vi "Mutate System Definition Driver VI And Dependency Paths.vi"(8 "error in (no error)":errorcluster, 11 "Section Ref in":T1 format="%.0x") -> (0 "error out":errorcluster, 3 "Section Ref out":T1 format="%.0x")   [LabVIEW 2019, in "Instrument Addon System Explorer.lvlib"]
uses:
  Instrument Addon System Explorer.lvlib
  <vilib>/NI VeriStand/Custom Device API/Path Type.ctl
  <vilib>/NI VeriStand/Custom Device API/Custom Device API.lvlib
  <vilib>/NI VeriStand/Custom Device API/Path Specification.ctl
  <vilib>/NI VeriStand/Custom Device API/Custom Device Supported Target.ctl
  <vilib>/NI VeriStand/Custom Device API/Custom Device Path Data.ctl
  NationalInstruments.VeriStand.SystemDefinitionAPI
  <vilib>/NI VeriStand/Custom Device API/Custom Device Item Ref.ctl
panel:
  in  "Current Version":string
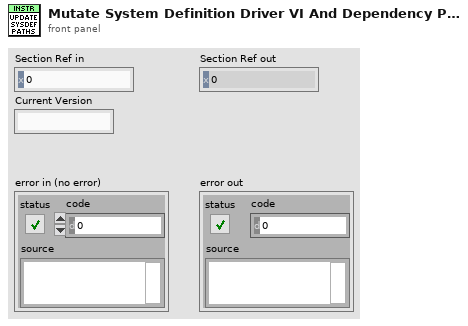
[diagram p1: front panel]
types:
  T1 = typedef "Custom Device API.lvlib/Custom Device Item Ref.ctl" = u64
  T2 = typedef "Custom Device API.lvlib/Custom Device Path Data.ctl" = cluster{"SupportedTarget":T3, "Source":T4, "RT Destination":path}
  T3 = typedef "Custom Device API.lvlib/Custom Device Supported Target.ctl" = enum16{"All", "PharLap", "VxWorks", "Windows", "Linux_32_ARM", "Linux_x64", "PharLap & Windows", "PharLap & VxWorks", "VxWorks & Windows"}
  T4 = typedef "Custom Device API.lvlib/Path Specification.ctl" = cluster{"Path":path, "Type":T5}
  T5 = typedef "Custom Device API.lvlib/Path Type.ctl" = enum16{"Absolute", "To Base", "To Common Data Dir", "To Application Data Dir"}
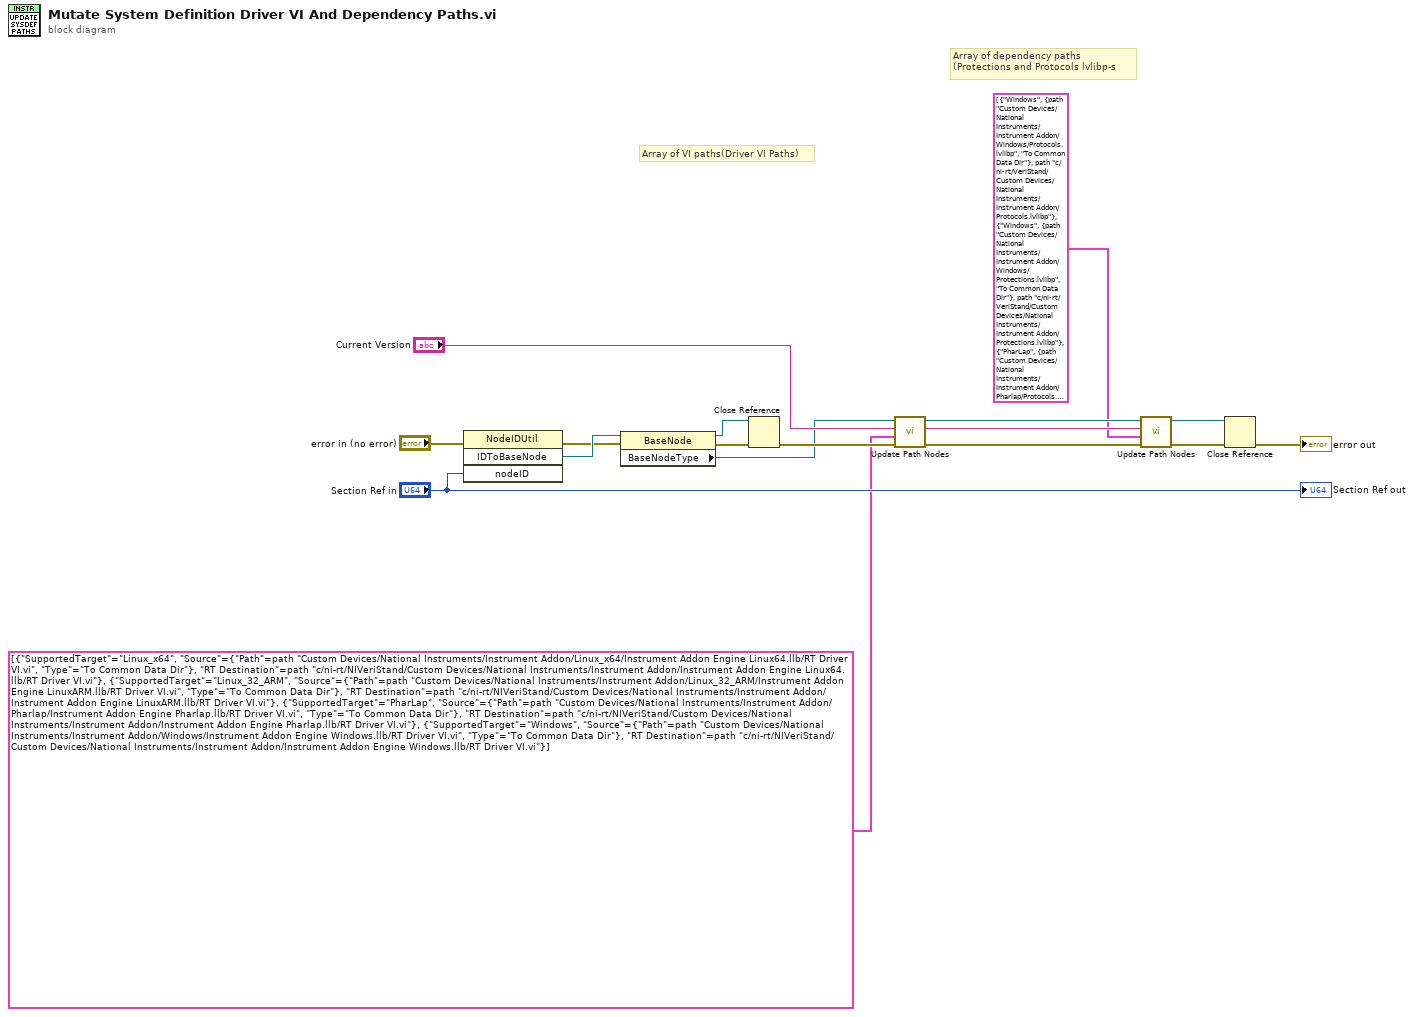
[diagram p0: block diagram]
diagram:
  # "Array of dependency paths\n(Protections and Protocols lvlibp-s"
  # "Array of VI paths(Driver VI Paths)"
  n1 = invoke class="NodeIDUtil" method="IDToBaseNode"(error in="error in (no error)", "nodeID"="Section Ref in") -> (error out=w11:errorcluster, "IDToBaseNode"=w12:refnum<k24>)  [unwired: 2 in, 2 out]
  n2 = property class="BaseNode"(reference=w12, error in=w11) -> (reference out=w14:refnum<k24>, error out=w13:errorcluster, "BaseNodeType"=w8:refnum<k24>)
  n3 = Close Reference(reference=w14, error in (no error)=w13) -> (error out=w16:errorcluster)
  n4 = call "Update Path Nodes.vi"("error in (no error)"=w16, "New Paths Array"=T2[] [{"SupportedTarget"=enum."Linux_x64", "Source"={"Path"=path "Custom Devices/National Instruments/Instrument Addon/Linux_x64/Instrument Addon Engine Linux64.llb/RT Driver VI.vi", "Type"=enum."To Common Data Dir"}, "RT Destination"=path "c:/ni-rt/NIVeriStand/Custom Devices/National Instruments/Instrument Addon/Instrument Addon Engine Linux64.llb/RT Driver VI.vi"}, {"SupportedTarget"=enum."Linux_32_ARM", "Source"={"Path"=path "Custom Devices/National Instruments/Instrument Addon/Linux_32_ARM/Instrument Addon Engine LinuxARM.llb/RT Driver VI.vi", "Type"=enum."To Common Data Dir"}, "RT Destination"=path "c:/ni-rt/NIVeriStand/Custom Devices/National Instruments/Instrument Addon/Instrument Addon Engine LinuxARM.llb/RT Driver VI.vi"}, {"SupportedTarget"=enum."PharLap", "Source"={"Path"=path "Custom Devices/National Instruments/Instrument Addon/Pharlap/Instrument Addon Engine Pharlap.llb/RT Driver VI.vi", "Type"=enum."To Common Data Dir"}, "RT Destination"=path "c:/ni-rt/NIVeriStand/Custom Devices/National Instruments/Instrument Addon/Instrument Addon Engine Pharlap.llb/RT Driver VI.vi"}, {"SupportedTarget"=enum."Windows", "Source"={"Path"=path "Custom Devices/National Instruments/Instrument Addon/Windows/Instrument Addon Engine Windows.llb/RT Driver VI.vi", "Type"=enum."To Common Data Dir"}, "RT Destination"=path "c:/ni-rt/NIVeriStand/Custom Devices/National Instruments/Instrument Addon/Instrument Addon Engine Windows.llb/RT Driver VI.vi"}] ("Driver VIs"), "Current Version in"="Current Version", ".NET Refnum in"=w8) -> ("error out"=w6:errorcluster, "Current Version out"=w5:string, ".NET Refnum out"=w7:refnum<k24>)  [unwired: 5 in]
  n5 = call "Update Path Nodes.vi"("error in (no error)"=w6, "New Paths Array"=T2[] [{"SupportedTarget"=enum."Windows", "Source"={"Path"=path "Custom Devices/National Instruments/Instrument Addon/Windows/Protocols.lvlibp", "Type"=enum."To Common Data Dir"}, "RT Destination"=path "c:/ni-rt/VeriStand/Custom Devices/National Instruments/Instrument Addon/Protocols.lvlibp"}, {"SupportedTarget"=enum."Windows", "Source"={"Path"=path "Custom Devices/National Instruments/Instrument Addon/Windows/Protections.lvlibp", "Type"=enum."To Common Data Dir"}, "RT Destination"=path "c:/ni-rt/VeriStand/Custom Devices/National Instruments/Instrument Addon/Protections.lvlibp"}, {"SupportedTarget"=enum."PharLap", "Source"={"Path"=path "Custom Devices/National Instruments/Instrument Addon/Pharlap/Protocols.lvlibp", "Type"=enum."To Common Data Dir"}, "RT Destination"=path "c:/ni-rt/VeriStand/Custom Devices/National Instruments/Instrument Addon/Protocols.lvlibp"}, {"SupportedTarget"=enum."PharLap", "Source"={"Path"=path "Custom Devices/National Instruments/Instrument Addon/Pharlap/Protections.lvlibp", "Type"=enum."To Common Data Dir"}, "RT Destination"=path "c:/ni-rt/VeriStand/Custom Devices/National Instruments/Instrument Addon/Protections.lvlibp"}, {"SupportedTarget"=enum."Linux_x64", "Source"={"Path"=path "Custom Devices/National Instruments/Instrument Addon/Linux_x64/Protocols.lvlibp", "Type"=enum."To Common Data Dir"}, "RT Destination"=path "c:/ni-rt/VeriStand/Custom Devices/National Instruments/Instrument Addon/Protocols.lvlibp"}, {"SupportedTarget"=enum."Linux_x64", "Source"={"Path"=path "Custom Devices/National Instruments/Instrument Addon/Linux_x64/Protections.lvlibp", "Type"=enum."To Common Data Dir"}, "RT Destination"=path "c:/ni-rt/VeriStand/Custom Devices/National Instruments/Instrument Addon/Protections.lvlibp"}, {"SupportedTarget"=enum."Linux_32_ARM", "Source"={"Path"=path "Custom Devices/National Instruments/Instrument Addon/Linux_32_ARM/Protocols.lvlibp", "Type"=enum."To Common Data Dir"}, "RT Destination"=path "c:/ni-rt/VeriStand/Custom Devices/National Instruments/Instrument Addon/Protocols.lvlibp"}, {"SupportedTarget"=enum."Linux_32_ARM", "Source"={"Path"=path "Custom Devices/National Instruments/Instrument Addon/Linux_32_ARM/Protections.lvlibp", "Type"=enum."To Common Data Dir"}, "RT Destination"=path "c:/ni-rt/VeriStand/Custom Devices/National Instruments/Instrument Addon/Protections.lvlibp"}] ("Depndencies"), "Current Version in"=w5, ".NET Refnum in"=w7) -> ("error out"=w3:errorcluster, ".NET Refnum out"=w2:refnum<k24>)  [unwired: 5 in, 1 out]
  n6 = Close Reference(reference=w2, error in (no error)=w3) -> (error out=→"error out":errorcluster)
  "Section Ref out" <- "Section Ref in"
